vi "BRig_comm_webdav__myrioAddress.vi"() -> (2 "output_myrioAddress":string="http://172.22.11.1")   [LabVIEW 2014]
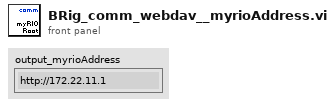
[diagram p1: front panel]
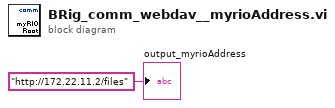
[diagram p0: block diagram]
diagram:
  "output_myrioAddress" <- "http://172.22.11.2/files" ("host uri prefix")
